vi "NI_9222_Anologue_DAQ3_FPGA.vi"() -> ()   [LabVIEW 2013]
uses:
  <vilib>/rvi/eio/common/nirviEmuClasses.ctl
  <vilib>/rvi/eio/common/nirviEmuTemplateMethod_errors.vi
  <vilib>/rvi/Emulation/niFpgaSctlEmulationGetInTimedLoop.vi
  <vilib>/rvi/Emulation/niFpgaEmulationReportErrorSimple.vi
  <vilib>/rvi/Emulation/niFpgaGetClockAttributes.vi
  <vilib>/rvi/Emulation/niFpgaProcessEmulError.vi
  <vilib>/rvi/Emulation/niFpgaCriticalErrorInLSC.vi
  <vilib>/rvi/interface/RandomDataEmulation/nirviRandomDataFPGAFIFO.vi
  <vilib>/rvi/interface/RandomDataEmulation/niFpgaRandomDataHandleErrors.vi
  <vilib>/eio/EIOGrowableMethodNode/genericMethod/EIOGrowableMethodNode.xnode
  <vilib>/rvi/eio/nirviEIOMethodImplementation/nirviEIOMethodImplementation.xnode
  <vilib>/rvi/eio/nirviErrorMerge/nirviErrorMerge.xnode
  <vilib>/rvi/DataTransferAndStorage/Container/XNode/niFpgaContainer.xnode
  <vilib>/rvi/interface/RandomDataEmulation/nirviRandomDataFpgaReadWriteTemplate.vi
panel:
  in  "Sample Period (uSec)":u32=2
  out "Timed Out":bool
  out "Overwrite":bool
  out "Sample Gated":bool
  out "Stopped":bool
  out "Error Out":errorcluster
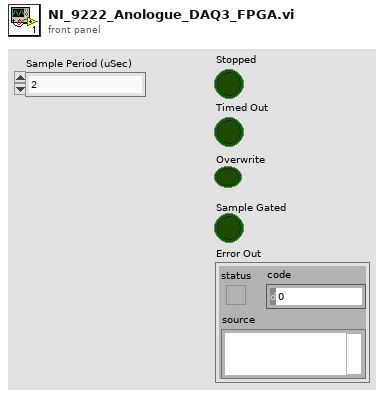
[diagram p1: front panel]
types:
  T1 = typedef "nirviEmuClasses.ctl" = enum16{"IO Read", "IO Write", "Method", "Property Read", "Property Write"}
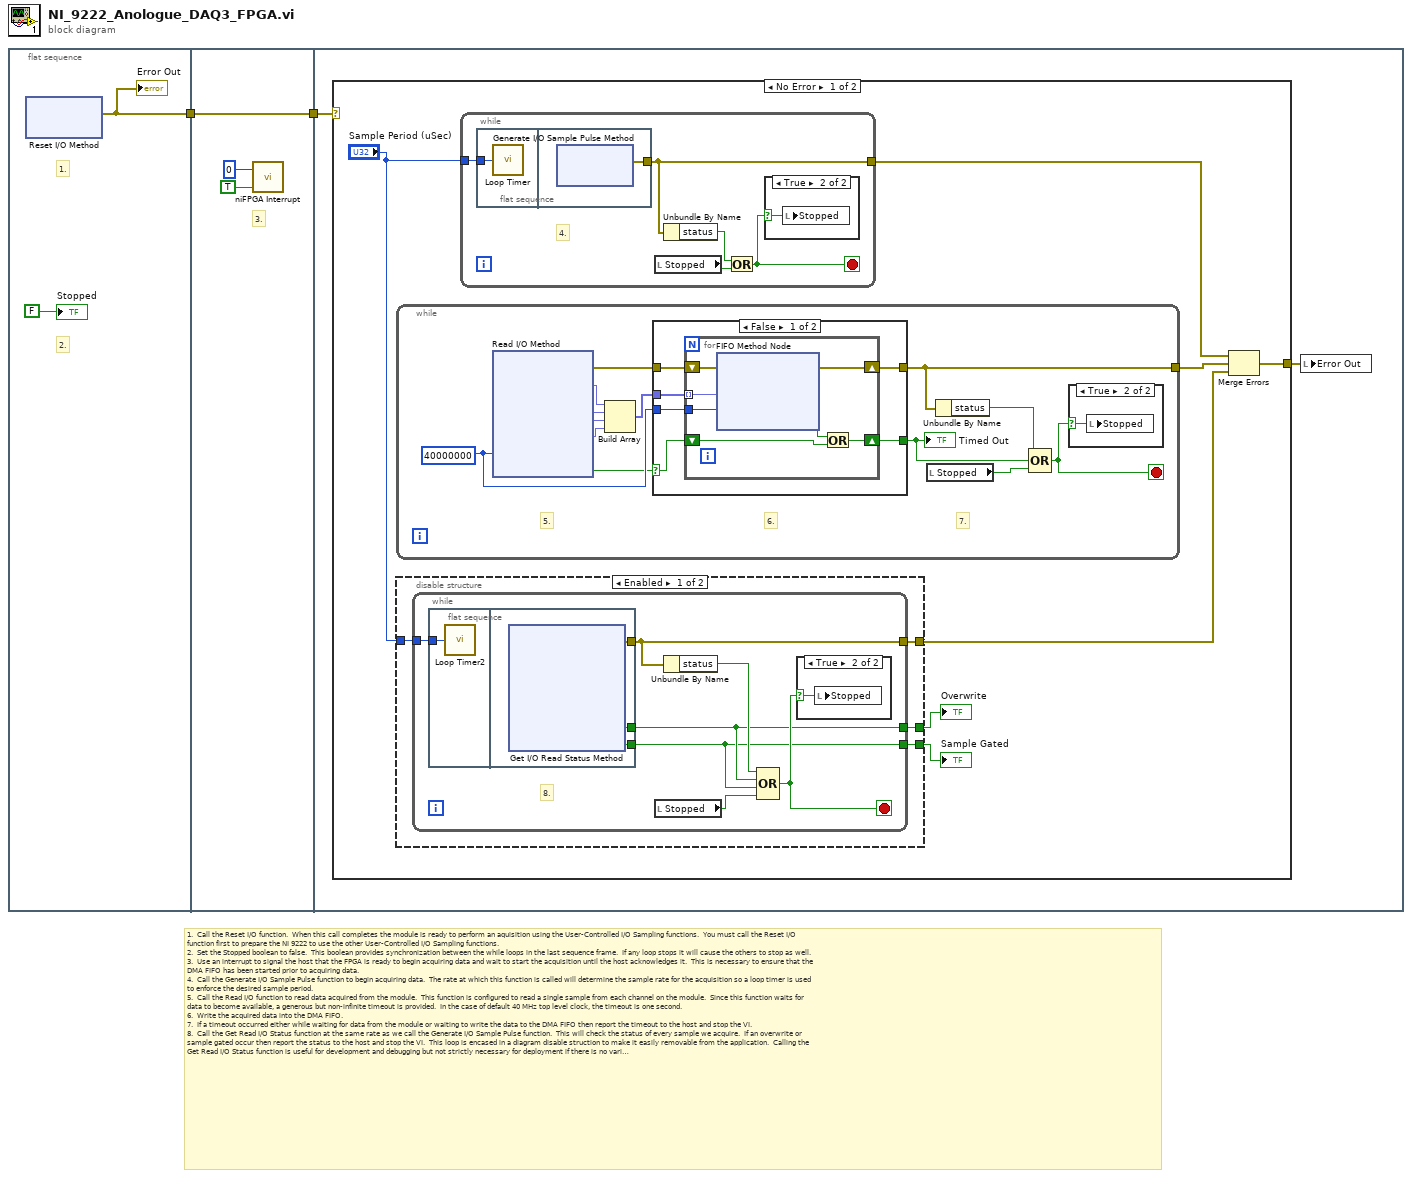
[diagram p0: block diagram]
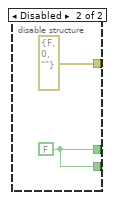
[diagram p3: hidden frame]
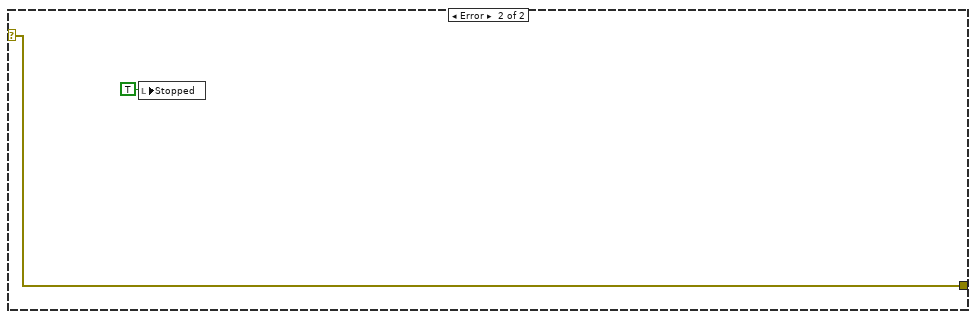
[diagram p7: hidden frame]
diagram:
  # "1.  Call the Reset I/O function.  When this call completes the module is ready to perform an aquisition using the User-Controlled I/O Sampling functions.  You must call the Reset I/O \nfunction first to prepare the NI 9222 to use the other User-Controlled I/O Sampling functions.\n2.  Set the Stopped boolean to false.  This boolean provides synchronization between the while loops in the last sequence frame.  If any loop stops it will cause the others to stop as well.\n3.  Use an interrupt to signal the host that the FPGA is ready to begin acquiring data and wait to start the acquisition until the host acknowledges it.  This is necessary to ensure that the \nDMA FIFO has been started prior to acquiring data.\n4.  Call the Generate I/O Sample Pulse function to begin acquiring data.  The rate at which this function is called will determine the sample rate for the acquisition so a loop timer is used\nto enforce the desired sample period.\n5.  Call the Read I/O function to read data acquired from the module.  This function is configured to read a single sample from each channel on the module.  Since this function waits for\ndata to become available, a generous but non-infinite timeout is provided.  In the case of default 40 MHz top level clock, the timeout is one second.\n6.  Write the acquired data into the DMA FIFO.\n7.  If a timeout occurred either while waiting for data from the module or waiting to write the data to the DMA FIFO then report the timeout to the host and stop the VI.\n8.  Call the Get Read I/O Status function at the same rate as we call the Generate I/O Sample Pulse function.  This will check the status of every sample we acquire.  If an overwrite or \nsample gated occur then report the status to the host and stop the VI.  This loop is encased in a diagram disable struction to make it easily removable from the application.  Calling the \nGet Read I/O Status function is useful for development and debugging but not strictly necessary for deployment if there is no variable timing in the application.  In the above example, it\nis not possible to get a sample gated status unless the top loop's sample period is less than the minimum sample period supported by the module.  However, this application could \nproduce an overwrite status if the host VI cannot read from the DMA FIFO fast enough."
  n1 = flat-sequence {
    tunnel: [w3] -> w2
    tunnel: w2 -> [w49]
    tunnel: [w49] -> w1
    tunnel: w1 -> [w53]
    frame #0 {
      # "2."
      # "1."
      n2 = xnode "Reset I/O Method"() -> ("error out"=w3:errorcluster)  [unwired: 2 in, 1 out]
      "Error Out" <- w3
      "Stopped" <- FALSE ("Stopped")
    }
    frame #1 {
      # "3."
      n3 = call <vilib>:"niFPGA Interrupt.vi"("Wait Until Cleared (F)"=TRUE ("Wait Until Cleared"), "IRQ Number (0)"=u8 0 ("IRQ Number")) -> ()  [unwired: 1 in]
    }
    frame #2 {
      n4 = case shown="No Error" w53 {
        selector: w53 -> [_ w508]
        tunnel: [w57 w508] -> w52
        frame No Error {
          n5 = while {
            tunnel: [w253] -> w59
            stop <- w248 stop-if-true
            w254 = 40000000 ("Timeout")
            # "7."
            # "6."
            # "5."
            n6 = xnode "Read I/O Method"("Timeout"=w254) -> ("error out"=w252:errorcluster, "Mod1/AI0"=w259:fxp<+/-,24,5>, "Mod1/AI1"=w258:fxp<+/-,24,5>, "Mod1/AI2"=w257:fxp<+/-,24,5>, "Mod1/AI3"=w256:fxp<+/-,24,5>, "Timed Out"=w251:bool)  [unwired: 5 in, 4 out]
            n7 = Build Array(w259, w258, w257, w256) -> (w255:fxp<+/-,24,5>[])
            n8 = case shown="False" w251 {
              selector: w251 -> [w261 w274]
              tunnel: w255 -> [w266 _]
              tunnel: w254 -> [w265 _]
              tunnel: [w264 w275] -> w253
              tunnel: [w263 w274] -> w247
              tunnel: w252 -> [w262 w275]
              frame False {
                n9 = for {
                  tunnel: w266 -> [w271] mode=indexing
                  shift-right: [w272] -> w264
                  shift-left: w262 -> [w273]
                  tunnel: w265 -> [w270]
                  shift-right: [w268] -> w263
                  shift-left: w261 -> [w267]
                  n10 = xnode ("FIFO Method Node")("Element"=w271, "Timeout"=w270, "error in (no error)"=w273) -> ("Timed Out?"=w269:bool, "error out"=w272:errorcluster)  [unwired: 1 in, 1 out]
                  n11 = Or(x=w269, y=w267) -> (x .or. y?=w268:bool)
                }
              }
              frame True {
              }
            }
            "Timed Out" <- w247
            n12 = local read "Stopped"() -> (w250:bool)
            n13 = Unbundle By Name(w253) -> ("status"=w249:bool)
            n14 = Compound Arithmetic op=OR(w249, w247, w250) -> (w248:bool)
            n15 = case shown="True" w248 {
              selector: w248 -> [_ w260]
              frame False {
              }
              frame True {
                n16 = local write "Stopped"(w260) -> ()
              }
            }
          }
          n17 = disable-structure shown="Enabled" {
            disable-tunnel: [w64 errorcluster {"status"=FALSE, "code"=0, "source"=""} ("error out")] -> w58
            disable-tunnel: "Sample Period (uSec)" -> [w63 _]
            disable-tunnel: [w62 w245] -> w55
            disable-tunnel: [w61 w245] -> w54
            frame Enabled {
              n18 = while {
                tunnel: [w71] -> w64
                tunnel: w63 -> [w70]
                tunnel: [w66] -> w62
                tunnel: [w65] -> w61
                stop <- w67 stop-if-true
                # "8."
                n19 = flat-sequence {
                  tunnel: w70 -> [w73]
                  tunnel: [w76] -> w71
                  tunnel: [w75] -> w66
                  tunnel: [w74] -> w65
                  frame #0 {
                    n20 = call "Loop Timer2"("Count(uSec)"=w73) -> ()  [unwired: 1 out]
                  }
                  frame #1 {
                    n21 = xnode "Get I/O Read Status Method"() -> ("error out"=w76:errorcluster, "Overwrite"=w75:bool, "Sample Gated"=w74:bool)  [unwired: 5 in, 4 out]
                  }
                }
                n22 = local read "Stopped"() -> (w69:bool)
                n23 = Unbundle By Name(w71) -> ("status"=w68:bool)
                n24 = Compound Arithmetic op=OR(w68, w66, w65, w69) -> (w67:bool)
                n25 = case shown="True" w67 {
                  selector: w67 -> [_ w72]
                  frame False {
                  }
                  frame True {
                    n26 = local write "Stopped"(w72) -> ()
                  }
                }
              }
            }
            frame Disabled {
              w245 = FALSE ("Overwrite")
            }
          }
          "Overwrite" <- w55
          "Sample Gated" <- w54
          n27 = while {
            tunnel: "Sample Period (uSec)" -> [w460]
            tunnel: [w457] -> w60
            stop <- w456 stop-if-true
            # "4."
            n28 = flat-sequence {
              tunnel: w460 -> [w462]
              tunnel: [w463] -> w457
              frame #0 {
                n29 = call "Loop Timer"("Count(uSec)"=w462) -> ()  [unwired: 1 out]
              }
              frame #1 {
                n30 = xnode "Generate I/O Sample Pulse Method"() -> ("error out"=w463:errorcluster)  [unwired: 2 in, 1 out]
              }
            }
            n31 = local read "Stopped"() -> (w459:bool)
            n32 = Unbundle By Name(w457) -> ("status"=w458:bool)
            n33 = Or(x=w458, y=w459) -> (x .or. y?=w456:bool)
            n34 = case shown="True" w456 {
              selector: w456 -> [_ w461]
              frame False {
              }
              frame True {
                n35 = local write "Stopped"(w461) -> ()
              }
            }
          }
          n36 = Merge Errors(w60, w59, w58) -> (w57:errorcluster)
        }
        frame Error {
          n37 = local write "Stopped"(TRUE ("Stopped")) -> ()
        }
      }
      n38 = local write "Error Out"(w52) -> ()
    }
  }
